vi "Alarm_Limit.vi"(7 "Alarm On":bool, 8 "Yellow Limit":dbl, 9 "Red Limit":dbl, 10 "Target":dbl format="%0.2f", 11 "Reading":dbl format="%0.2f") -> (2 "Alarm Output":bool[](array[boolean]))   [LabVIEW 2014]
panel:
  # "Alarm Indicator"
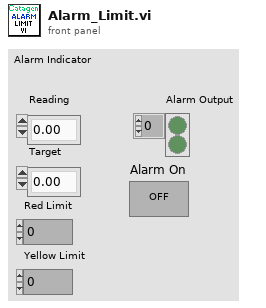
[diagram p1: front panel]
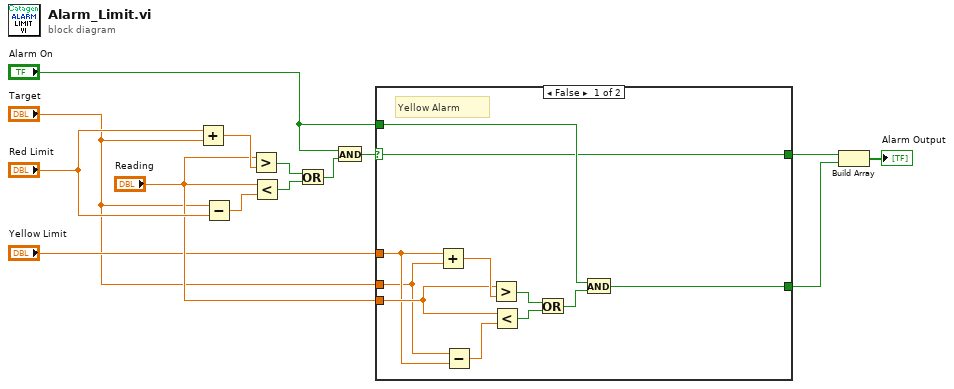
[diagram p0: block diagram]
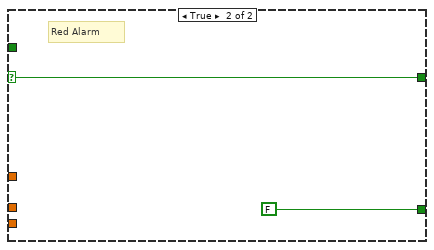
[diagram p2: hidden frame]
diagram:
  n1 = Add(x="Red Limit", y="Target") -> (x+y=w13:dbl)
  n2 = Subtract(x="Target", y="Red Limit") -> (x-y=w12:dbl)
  n3 = Greater?(x="Reading", y=w13) -> (0:w10:bool)
  n4 = Less?(x="Reading", y=w12) -> (x < y?=w9:bool)
  n5 = Or(x=w10, y=w9) -> (x .or. y?=w11:bool)
  n6 = And(x="Alarm On", y=w11) -> (x .and. y?=w8:bool)
  n7 = case shown="False" w8 {
    selector: w8 -> [w16 w27]
    tunnel: "Reading" -> [w21 _]
    tunnel: "Yellow Limit" -> [w20 _]
    tunnel: "Alarm On" -> [w18 _]
    tunnel: [w17 FALSE] -> w2
    tunnel: [w16 w27] -> w3
    tunnel: "Target" -> [w15 _]
    frame False {
      # "Yellow Alarm"
      n8 = Add(x=w20, y=w15) -> (x+y=w22:dbl)
      n9 = Subtract(x=w15, y=w20) -> (x-y=w23:dbl)
      n10 = Greater?(x=w21, y=w22) -> (0:w24:bool)
      n11 = Less?(x=w21, y=w23) -> (x < y?=w25:bool)
      n12 = Or(x=w24, y=w25) -> (x .or. y?=w19:bool)
      n13 = And(x=w18, y=w19) -> (x .and. y?=w17:bool)
    }
    frame True {
      # "Red Alarm"
    }
  }
  n14 = Build Array(w3, w2) -> (→"Alarm Output":bool[])
